vi "analogica.vi"() -> ()   [LabVIEW 2016]
panel:
  out "data":dynamicdata(graph)
  in  "stop (F)":bool
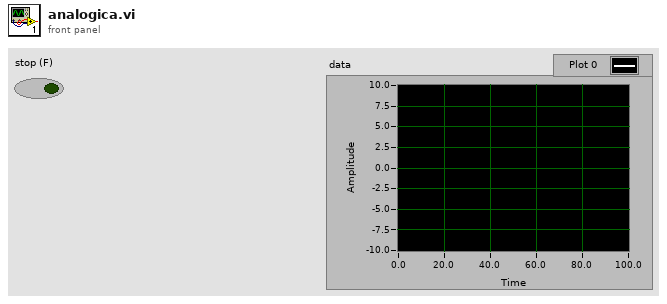
[diagram p1: front panel]
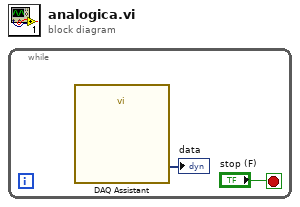
[diagram p0: block diagram]
diagram:
  n1 = while {
    stop <- "stop (F)" stop-if-true
    n2 = call "DAQ Assistant"() -> ("data"=→"data":dynamicdata)  [unwired: 16 in, 3 out]
  }
